vi "max and min values of an array.vi"() -> ()   [LabVIEW 2025]
panel:
  out "min index":dbl
  out "max index":dbl
  out "min number":dbl
  out "max number":dbl
  in  "Array":dbl[](array[numeric])
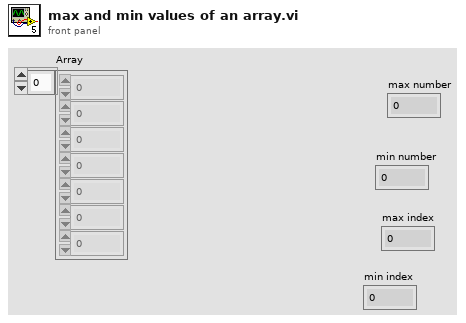
[diagram p1: front panel]
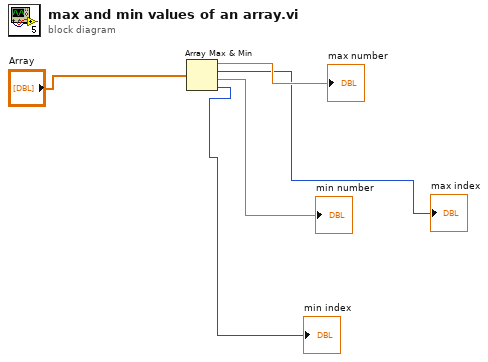
[diagram p0: block diagram]
diagram:
  n1 = Array Max & Min(array="Array") -> (max value=→"max number":dbl, max index (indices)=→"max index":i32, min value=→"min number":dbl, min index (indices)=→"min index":i32)
